vi "align PZT center.vi"(8 "error in":errorcluster, 11 "Coarse Approach in":refnum<class "Coarse Approach.lvclass">) -> (0 "error out":errorcluster, 3 "Coarse Approach out":refnum<class "Coarse Approach.lvclass">)   [LabVIEW 2020, in "Coarse Approach.lvclass"]
uses:
  Coarse Approach.lvclass
  Coarse Approach.lvclass/Coarse Approach.ctl
  PZT/PZT.lvclass
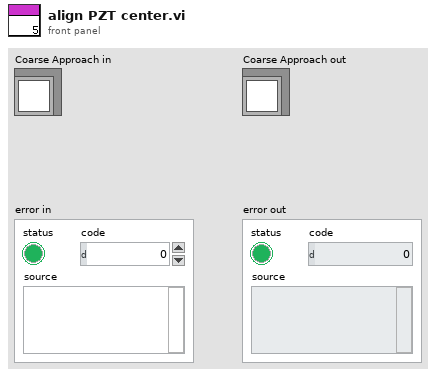
[diagram p1: front panel]
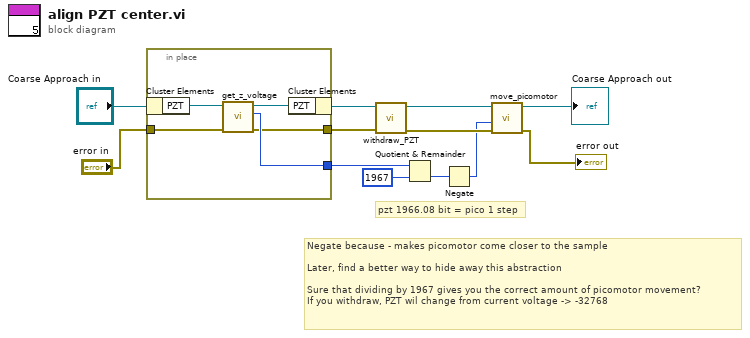
[diagram p0: block diagram]
diagram:
  # "Negate because - makes picomotor come closer to the sample\n\nLater, find a better way to hide away this abstraction\n\nSure that dividing by 1967 gives you the correct amount of picomotor movement?\nIf you withdraw, PZT wil change from current voltage -> -32768"
  # "pzt 1966.08 bit = pico 1 step"
  n1 = in-place {
    in-place-border: [w15] -> w11
    in-place-border: "error in" -> [w14]
    in-place-border: [w13] -> w4
    n2 = in-place-cluster #1("Coarse Approach in") -> ("PZT"=w17:refnum<class "PZT.lvclass">)
    n3 = call "get_z_voltage.vi"("error in"=w14, "PZT in"=w17) -> ("error out"=w13:errorcluster, "Z Voltage out"=w15:i16, "PZT out"=w16:refnum<class "PZT.lvclass">)  [unwired: 7 in]
    n4 = in-place-cluster #1("PZT"=w16) -> (w9:refnum<class "Coarse Approach.lvclass">)
  }
  n5 = call "withdraw_PZT.vi"("error in"=w4, "Coarse Approach in"=w9) -> ("error out"=w7:errorcluster, "Coarse Approach out"=w8:refnum<class "Coarse Approach.lvclass">)  [unwired: 8 in]
  n6 = Quotient & Remainder(x=w11, y=i16 1967) -> (floor(x/y)=w2:i16)  [unwired: 1 out]
  n7 = Negate(x=w2) -> (-x=w1:i16)
  n8 = call "move_picomotor.vi"("error in"=w7, "Destination (steps)"=w1, "Coarse Approach in"=w8) -> ("error out"=→"error out":errorcluster, "Coarse Approach out"=→"Coarse Approach out":refnum<class "Coarse Approach.lvclass">)  [unwired: 6 in, 1 out]
